vi "Get Scheduled Tx Execution Time.vi"(8 "error in":errorcluster, 11 "timing ref":T1=18446744073709551615 format="%.0x") -> (0 "error out":errorcluster, 2 "sched tx execution time ref":T1 format="%.0x", 3 "timing ref out":T1 format="%.0x")   [LabVIEW 2020, in "AIM ARINC 429 Scripting.lvlib"]
doc: "Returns true if logging is enabled."
uses:
  AIM ARINC 429 Scripting.lvlib
  Constants.vi
  <vilib>/NI VeriStand/Custom Device Tools/Custom Device Utility Library/Custom Device Utility Library.lvlib
  <vilib>/NI VeriStand/Custom Device Tools/Custom Device Utility Library/NI VeriStand - Search for Item by Name.vi
  <vilib>/NI VeriStand/Custom Device API/Custom Device Item Ref.ctl
  <vilib>/NI VeriStand/Custom Device API/Custom Device API.lvlib
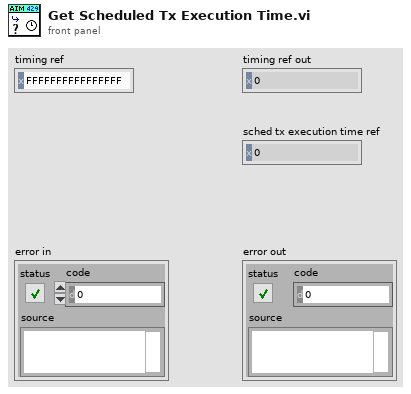
[diagram p1: front panel]
types:
  T1 = typedef "Custom Device API.lvlib/Custom Device Item Ref.ctl" = u64
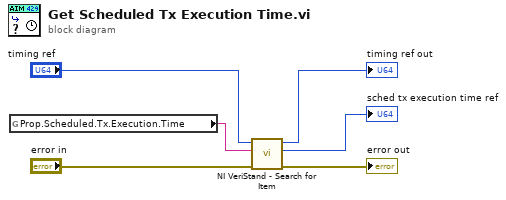
[diagram p0: block diagram]
diagram:
  n1 = global read "Constants.vi" "Prop.Scheduled.Tx.Execution.Time"() -> (w6:string)
  n2 = call-poly <vilib>:"NI VeriStand - Search for Item.vi"("error in"="error in", "Item Name"=w6, "Section Ref in"="timing ref") -> ("error out"=→"error out":errorcluster, "Item Ref"=→"sched tx execution time ref":T1, "Section Ref out"=→"timing ref out":T1)  [unwired: 5 in, 1 out]
